vi "Set Load Current.vi"(0 "instrument handle in":refnum<k15>, 1 "timeout (sec)":dbl=10.0, 5 "current level":dbl format="%.6p", 7 "OutputFunction":T1, 11 "error in (no error)":errorcluster) -> (4 "instrument handle out":refnum<k15>, 15 "error out":errorcluster)   [LabVIEW 2020]
uses:
  Load Output Function.ctl
  <instrlib>/niDCPower/nidcpower.llb/niDCPower Wait For Event - Event.ctl
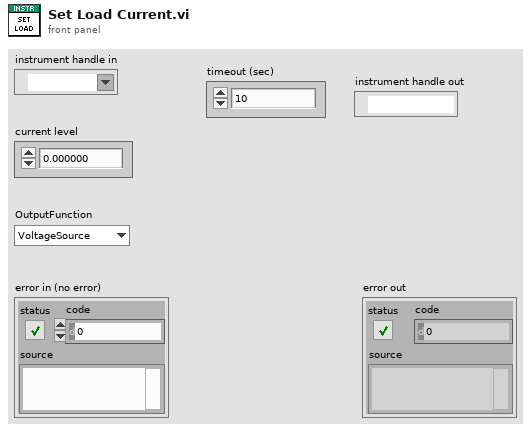
[diagram p1: front panel]
types:
  T1 = typedef "Load Output Function.ctl" = enum16{"VoltageSource", "CurrentSource"}
  T2 = typedef "niDCPower Wait For Event - Event.ctl" = i32
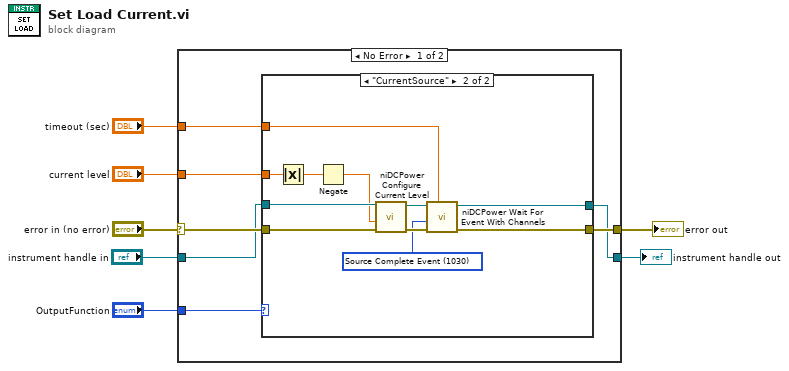
[diagram p0: block diagram]
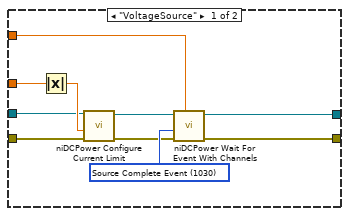
[diagram p2: hidden frame]
diagram:
  n1 = case shown="No Error" "error in (no error)" {
    selector: "error in (no error)" -> [w10 w37]
    tunnel: "OutputFunction" -> [w14 _]
    tunnel: [w13 w37] -> w5
    tunnel: "current level" -> [w12 _]
    tunnel: "timeout (sec)" -> [w11 _]
    tunnel: "instrument handle in" -> [w9 w36]
    tunnel: [w8 w36] -> w1
    frame No Error {
      n2 = case shown="\"CurrentSource\"" w14 {
        tunnel: [w18 w32] -> w13
        tunnel: w10 -> [w24 w31]
        tunnel: w9 -> [w21 w30]
        tunnel: w12 -> [w23 w29]
        tunnel: w11 -> [w16 w26]
        tunnel: [w15 w25] -> w8
        frame "VoltageSource" {
          w20 = T2 1030 items=["Source Complete Event"=1030, "Measure Complete Event"=1031, "Sequence Iteration Complete Event"=1032, "Sequence Engine Done Event"=1033, "Pulse Complete Event"=1051, "Ready For Pulse Trigger Event"=1052] ("event")
          n3 = Absolute Value(x=w23) -> (abs(x)=w22:dbl)
          n4 = call <instrlib>:"niDCPower Configure Current Limit.vi"("error in (no error)"=w24, "current limit"=w22, "instrument handle"=w21) -> ("error out"=w19:errorcluster, "instrument handle out"=w17:refnum<k15>)  [unwired: 7 in]
          n5 = call <instrlib>:"niDCPower Wait For Event With Channels.vi"("timeout (10.0)"=w16, "error in (no error)"=w19, "event"=w20, "instrument handle"=w17) -> ("error out"=w18:errorcluster, "instrument handle out"=w15:refnum<k15>)  [unwired: 6 in]
        }
        frame "CurrentSource" {
          w33 = T2 1030 items=["Source Complete Event"=1030, "Measure Complete Event"=1031, "Sequence Iteration Complete Event"=1032, "Sequence Engine Done Event"=1033, "Pulse Complete Event"=1051, "Ready For Pulse Trigger Event"=1052] ("event")
          n6 = Absolute Value(x=w29) -> (abs(x)=w28:dbl)
          n7 = Negate(x=w28) -> (-x=w27:dbl)
          n8 = call <instrlib>:"niDCPower Configure Current Level.vi"("error in (no error)"=w31, "current level"=w27, "instrument handle"=w30) -> ("error out"=w35:errorcluster, "instrument handle out"=w34:refnum<k15>)  [unwired: 7 in]
          n9 = call <instrlib>:"niDCPower Wait For Event With Channels.vi"("timeout (10.0)"=w26, "error in (no error)"=w35, "event"=w33, "instrument handle"=w34) -> ("error out"=w32:errorcluster, "instrument handle out"=w25:refnum<k15>)  [unwired: 6 in]
        }
      }
    }
    frame Error {
    }
  }
  "error out" <- w5
  "instrument handle out" <- w1
